vi "detachPos.vi"() -> ()   [LabVIEW 2014]
panel:
  out "error out":errorcluster
  in  "input string":string
  out "Z":dbl
  out "Y":dbl
  out "X":dbl
  # "String nhan tu UART co dang\nX:0.50 Y:0.00 Z:0.00 E:0.00"
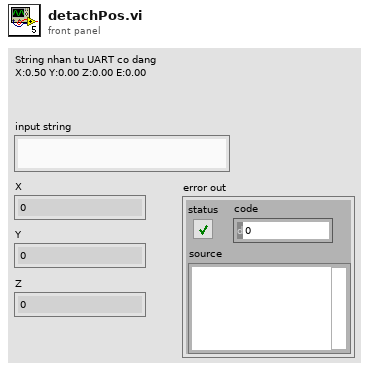
[diagram p1: front panel]
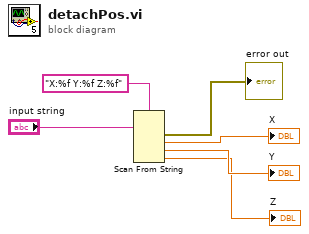
[diagram p0: block diagram]
diagram:
  n1 = Scan From String(format string="X:%f Y:%f Z:%f", input string="input string") -> (error out=→"error out":errorcluster, output 1=→"X":dbl, output 2=→"Y":dbl, output 3=→"Z":dbl)  [unwired: 5 in, 2 out]
